vi "Create.vi"(7 "_Rescript in":refnum<class "_Rescript.lvclass">, 8 "error in":errorcluster) -> (0 "error out":errorcluster, 5 "_Rescript out":refnum<class "_Rescript.lvclass">)   [LabVIEW 2025, in "_Rescript.lvlib" / "Msg.lvlib"]
uses:
  Msg.lvlib
  _Shared/Project Stuff/Project Stuff.lvclass
  _Shared/Name Specs/Name Specs.lvclass
  _Rescript/_Rescript.lvclass
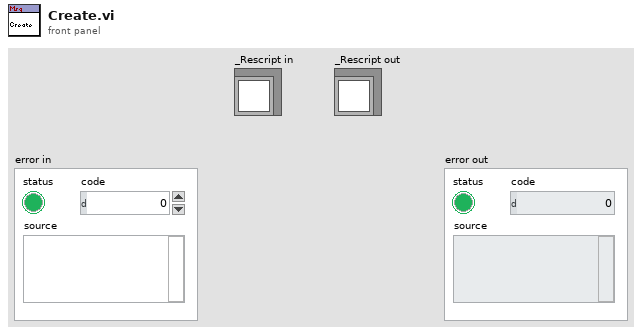
[diagram p1: front panel]
types:
  T1 = typedef "_Shared.lvlib/Name Stuff.ctl" = cluster{"Type (Enum)":T2, "Type (String)":string, "Name Library File Path":path, "Name":string, "Name Type":string}
  T2 = typedef "_Shared.lvlib/Type.ctl" = enum16{"Actor", "Msg"}
  T3 = typedef "_Rescript.lvlib/Msg.lvlib/Name jettl Msg.ctl" = cluster{"Name VI (Interface)":refnum<vi>}
  T4 = typedef "_Rescript.lvlib/Msg.lvlib/Name Msg.ctl" = cluster{"Execute VI (Class)":refnum<vi>}
  T5 = typedef "_Rescript.lvlib/Msg.lvlib/Name Msg Output.ctl" = cluster{"PD Control (Class)":refnum<vi>, "PD Cluster (Class)":refnum<vi>, "Init Msg Output VI (Class)":refnum<vi>, "Read Msg Output VI (Class)":refnum<vi>, "Init Msg Output VI (Lib)":refnum<vi>, "Read Msg Output VI (Lib)":refnum<vi>, "Terminal Attributes (Init)":T6, "Terminal Attributes (Read)":T6}
  T6 = typedef "_Rescript.lvlib/Terminal Attributes.ctl" = map{i32, T7}
  T7 = typedef "_Rescript.lvlib/Attributes.ctl" = cluster{"Control":refnum<vi>, "Wire Rule":enum16{"Invalid Wire Rule", "Required", "Recommended", "Optional", "Dynamic Dispatch"}}
  T8 = typedef "_Rescript.lvlib/Msg.lvlib/Name.ctl" = cluster{"Name VI (Lib)":refnum<vi>, "Init Msg VI (Lib)":refnum<vi>, "Call VI (Lib)":refnum<vi>, "Recurse VI (Lib)":refnum<vi>, "Tell Self VI (Lib)":refnum<vi>, "Tell Parent VI (Lib)":refnum<vi>, "Tell Child VI (Lib)":refnum<vi>, "Tell Reply VI (Lib)":refnum<vi>}
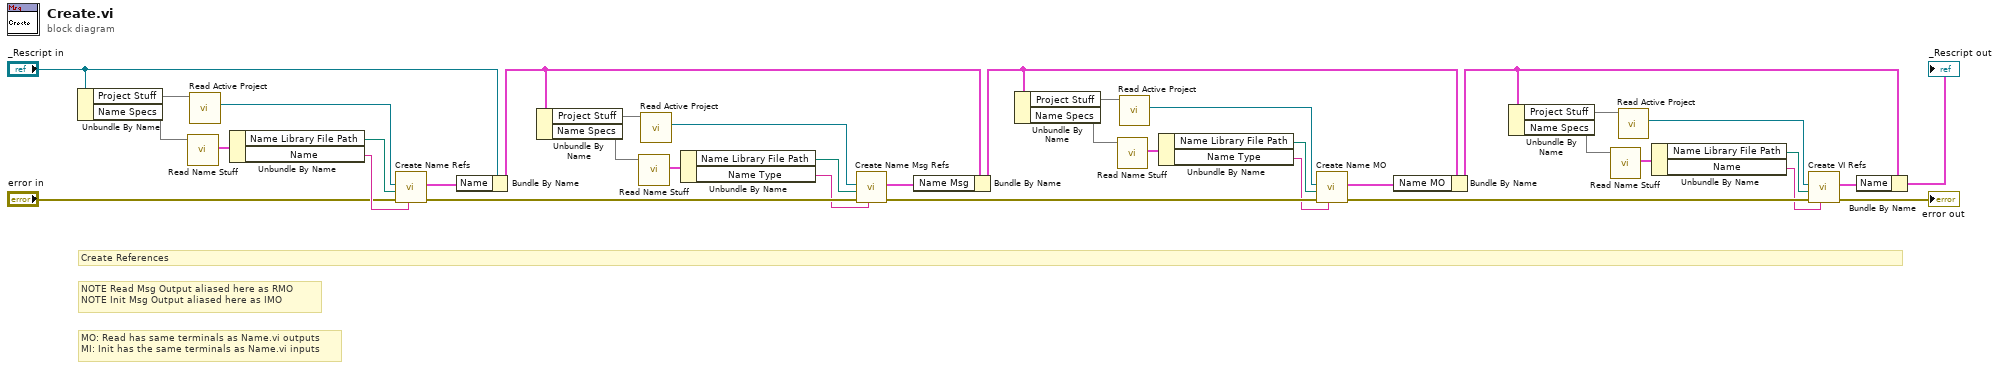
[diagram p0: block diagram]
diagram:
  # "MO: Read has same terminals as Name.vi outputs\nMI: Init has the same terminals as Name.vi inputs"
  # "NOTE Read Msg Output aliased here as RMO\nNOTE Init Msg Output aliased here as IMO"
  # "Create References"
  n1 = Unbundle By Name("_Rescript in") -> ("Project Stuff"=w10, "Name Specs"=w35)
  n2 = call "Read Name Stuff.vi"("Name Specs in"=w35) -> ("Name Stuff"=w34:T1)  [unwired: 10 in]
  n3 = call "Read Active Project.vi"("Project Stuff in"=w10) -> ("Active Project"=w9:refnum<vi>)  [unwired: 10 in]
  n4 = Unbundle By Name(w34) -> ("Name Library File Path"=w12:path, "Name"=w11:string)
  n5 = call "Create Name Refs.vi"("Name"=w11, "error in"="error in", "Name Library File Path"=w12, "Active Project"=w9) -> ("error out"=w38:errorcluster, "Name Refs"=w33:T3)  [unwired: 6 in]
  n6 = Bundle By Name(cluster="_Rescript in", "Name"=w33) -> (w30:cluster{})
  n7 = Unbundle By Name(w30) -> ("Project Stuff"=w29, "Name Specs"=w31)
  n8 = call "Read Name Stuff.vi"("Name Specs in"=w31) -> ("Name Stuff"=w32:T1)  [unwired: 10 in]
  n9 = call "Read Active Project.vi"("Project Stuff in"=w29) -> ("Active Project"=w28:refnum<vi>)  [unwired: 10 in]
  n10 = Unbundle By Name(w32) -> ("Name Library File Path"=w27:path, "Name Type"=w26:string)
  n11 = call "Create Name Msg Refs.vi"("Name Msg"=w26, "error in"=w38, "Name Library File Path"=w27, "Active Project"=w28) -> ("error out"=w37:errorcluster, "Name Msg Refs"=w25:T4)  [unwired: 6 in]
  n12 = Bundle By Name(cluster=w30, "Name Msg"=w25) -> (w21:cluster{})
  n13 = Unbundle By Name(w21) -> ("Project Stuff"=w24, "Name Specs"=w23)
  n14 = call "Read Name Stuff.vi"("Name Specs in"=w23) -> ("Name Stuff"=w22:T1)  [unwired: 10 in]
  n15 = call "Read Active Project.vi"("Project Stuff in"=w24) -> ("Active Project"=w20:refnum<vi>)  [unwired: 10 in]
  n16 = Unbundle By Name(w22) -> ("Name Library File Path"=w19:path, "Name Type"=w18:string)
  n17 = call "Create Name MO.vi"("Name Msg"=w18, "error in"=w37, "Name Library File Path"=w19, "Active Project"=w20) -> ("error out"=w36:errorcluster, "Name Msg Output Refs"=w17:T5)  [unwired: 6 in]
  n18 = Bundle By Name(cluster=w21, "Name MO"=w17) -> (w14:cluster{})
  n19 = Unbundle By Name(w14) -> ("Project Stuff"=w8, "Name Specs"=w16)
  n20 = call "Read Name Stuff.vi"("Name Specs in"=w16) -> ("Name Stuff"=w15:T1)  [unwired: 10 in]
  n21 = call "Read Active Project.vi"("Project Stuff in"=w8) -> ("Active Project"=w5:refnum<vi>)  [unwired: 10 in]
  n22 = Unbundle By Name(w15) -> ("Name Library File Path"=w6:path, "Name"=w7:string)
  n23 = call "Create VI Refs.vi"("Name"=w7, "error in"=w36, "Name Library File Path"=w6, "Active Project"=w5) -> ("error out"=→"error out":errorcluster, "VI Refs"=w13:T8)  [unwired: 6 in]
  n24 = Bundle By Name(cluster=w14, "Name"=w13) -> (→"_Rescript out":cluster{})
